vi "PH_PowerUnit_BaseClass.panel.vi"() -> ()   [LabVIEW 2014, in "PH_PowerUnit_BaseClass.lvlib"]
uses:
  PH_PowerUnit_BaseClass.lvlib
  PH_StatusHandler/PH_StatusHandler.GUI element.ctl
  PH_PowerUnit_BaseClass.GUI Refs to pack.ctl
  PH_PowerUnit_BaseClass.GUI Refs.ctl
  CSCore/CSObj/CSObj.lvlib
  PH_Common/PH_Common.lvlib
  PH_Class/PH_Class.lvlib
  PH_StatusHandler/PH_StatusHandler.lvlib
panel:
  out "Timing":u32(colorbox)=6618880
  in  "PU on":bool
  out "Seq SM State":string
  out "PSDB Status":u32(colorbox)=6618880 caption="PSDB"
  out "Dummy 2":u32(colorbox)=6618880
  out "Status":T1 caption="State PU"
  out "Dummy 1":u32(colorbox)=6618880
  in  "Exit":bool
  out "Waiting Time":dbl=999999.0
  out "error out":errorcluster
  in  "Delete":bool
  in  "error in (no error)":errorcluster
  in  "object ref":refnum<vi>
  out "Enabled":u32(colorbox)=6618880
  # "PCS"
  # "3.40"
  # "s"
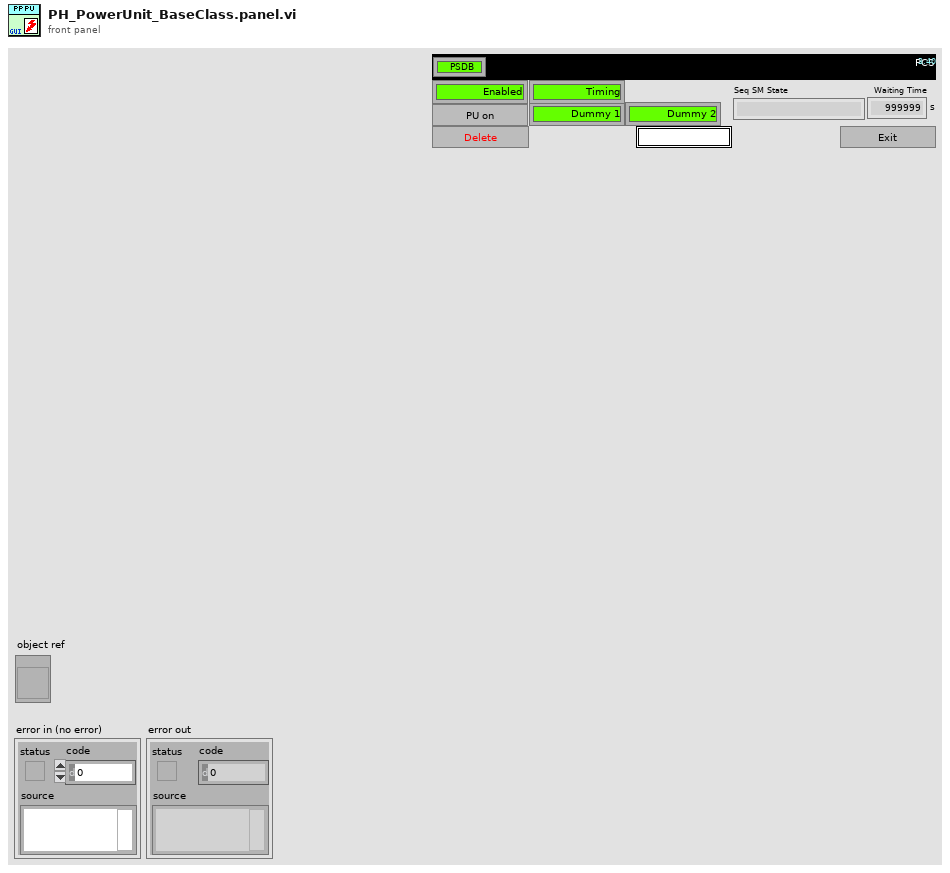
[diagram p1: front panel]
types:
  T1 = typedef "PH_StatusHandler.lvlib/PH_StatusHandler.GUI element.ctl" = u16
  T2 = typedef "PH_PowerUnit_BaseClass.lvlib/PH_PowerUnit_BaseClass.GUI Refs to pack.ctl" = cluster{"GUI Refs":T3, "Enabled":refnum<vi>, "PU on":refnum<vi>, "Waiting Time":refnum<vi>, "Timing.Instance":refnum<vi>, "Seq SM State":refnum<vi>, "Subscribed Trendmssgs":refnum<vi>[]}
  T3 = typedef "PH_PowerUnit_BaseClass.lvlib/PH_PowerUnit_BaseClass.GUI Refs.ctl" = cluster{"Delete Inst":refnum<vi>, "State TO SM":refnum<vi>, "State SM":refnum<vi>, "Fire":refnum<vi>}
  T4 = cluster{"GUI Refs Power Unit Base Class":T2, "PSDB Status":refnum<vi>}
  T5 = typedef "PH_PowerUnit_BaseClass.lvlib/PH_PowerUnit_BaseClass.i attribute.ctl" = cluster{"Constructor finished":bool, "PU":cluster{"In use":bool, "Service ID in use":i32, "GUI Ref":refnum<vi>}, "Enabling":cluster{"State":T6, "GUI Ref":refnum<vi>}, "Timing":cluster{"Last Shot":dbl, "Time between Shots [Sec]":dbl, "Waiting Time over?":bool, "Service ID Waiting Time":i32, "GUI Ref":refnum<vi>, "Instance":cluster{"Status":T7, "linked?":bool, "GUI Ref":refnum<vi>}}, "Sequencer":cluster{"SM State":string, "GUI Ref":refnum<vi>, "linked":bool}, "Subscribed Trendmssgs":cluster{"Tagname":string, "Status":T7, "linked?":bool, "Shot Condition":T7, "GUI Ref":refnum<vi>}[], "PP PU":T8, "Default Voltage (V)":dbl, "GUI Refs":T3, "PSDB data":cluster{"Shot Voltage [V]":dbl, "State TO SM":T9, "Write 2 early":bool}, "State TO SM":T9}
  T6 = typedef "PH_SystemInformation.lvlib/PH_SystemInformationEnabling State.ctl" = i32
  T7 = typedef "PH_StatusHandler.lvlib/PH_StatusHandler.Status.ctl" = i16
  T8 = typedef "PH_PP_Common.lvlib/PH_PP_Common.PUs.ctl" = enum16{"no Info", "PA-19mm-1", "PA-19mm-2", "PA-45mm-PILC", "PA-45mm-MAIN", "MA-PU-1", "MA-PU-2", "MA-PU-3", "MA-PU-4", "MA-PU-5", "MA-PU-6", "MA-FR", "MA-PILC", "PA-45mm-DP"}
  T9 = typedef "PH_PowerUnit_BaseClass.lvlib/PH_PowerUnit_BaseClass.SM States.ctl" = enum16{".", "Stand by", "Switch PU on", "Configure", "Set Default Voltage", "Set STANDBY", "Set READY", "Wait for Shot Cmd", "Open Dump Rods", "Open Ross Relais", "Close Ross Relais", "Switch PSU on", "Switch PSU off", "Charge", "Switch GD Channel on", "Close Dump Rods", "Rods-TO", "RR-TO", "PSU-TO", "Trigger-TO"}
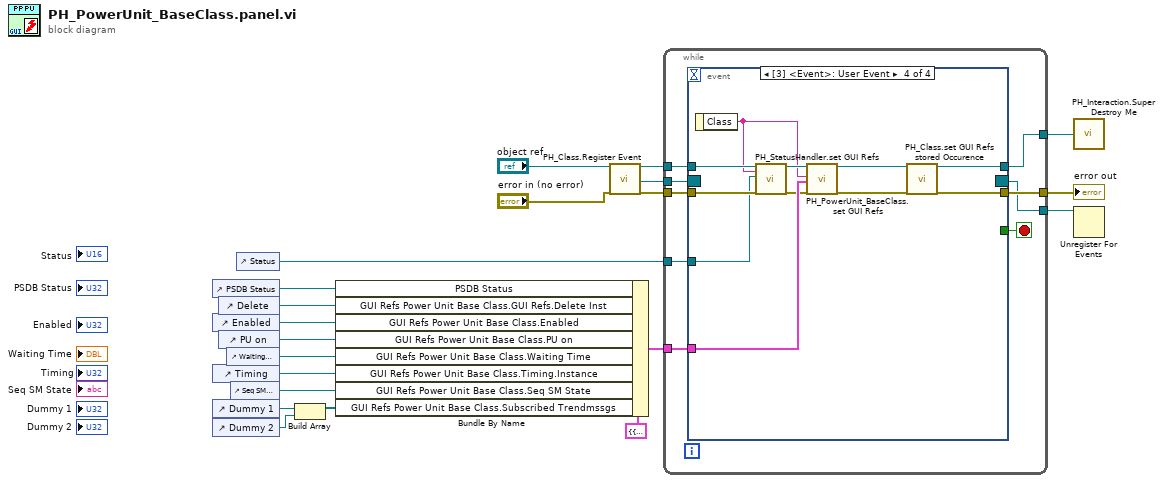
[diagram p0: block diagram]
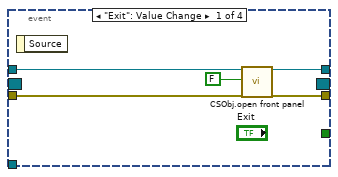
[diagram p2: hidden frame]
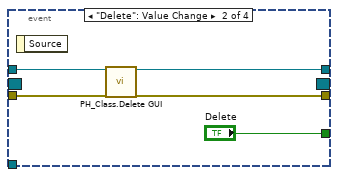
[diagram p3: hidden frame]
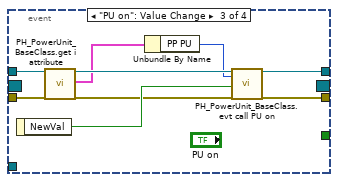
[diagram p4: hidden frame]
diagram:
  n1 = control-ref of="PSDB Status"() -> (w12:refnum<vi>)
  n2 = control-ref of="Enabled"() -> (w10:refnum<vi>)
  n3 = control-ref of="Timing"() -> (w7:refnum<vi>)
  n4 = control-ref of="Dummy 1"() -> (w19:refnum<vi>)
  n5 = control-ref of="Dummy 2"() -> (w18:refnum<vi>)
  n6 = control-ref of="Delete"() -> (w11:refnum<vi>)
  n7 = control-ref of="PU on"() -> (w9:refnum<vi>)
  n8 = control-ref of="Waiting Time"() -> (w8:refnum<vi>)
  n9 = control-ref of="Seq SM State"() -> (w6:refnum<vi>)
  n10 = control-ref of="Status"() -> (w1:refnum<vi>)
  n11 = Build Array(w19, w18) -> (w5:refnum<vi>[])
  n12 = Bundle By Name(cluster=T4 {"GUI Refs Power Unit Base Class"={"GUI Refs"={"Delete Inst"=refnum, "State TO SM"=refnum, "State SM"=refnum, "Fire"=refnum}, "Enabled"=refnum, "PU on"=refnum, "Waiting Time"=refnum, "Timing.Instance"=refnum, "Seq SM State"=refnum, "Subscribed Trendmssgs"=[]}, "PSDB Status"=refnum} ("GUI Refs"), "PSDB Status"=w12, "GUI Refs Power Unit Base Class.GUI Refs.Delete Inst"=w11, "GUI Refs Power Unit Base Class.Enabled"=w10, "GUI Refs Power Unit Base Class.PU on"=w9, "GUI Refs Power Unit Base Class.Waiting Time"=w8, "GUI Refs Power Unit Base Class.Timing.Instance"=w7, "GUI Refs Power Unit Base Class.Seq SM State"=w6, "GUI Refs Power Unit Base Class.Subscribed Trendmssgs"=w5) -> (w2:T4)
  n13 = call "PH_Class.Register Event.vi"("i ref in"="object ref", "error in (no error)"="error in (no error)") -> ("i ref out"=w17:refnum<vi>, "Event Registration Refnum"=w15:refnum<event-registration>, "error out"=w16:errorcluster)  [unwired: 15 in]
  n14 = while {
    tunnel: w17 -> [w27]
    tunnel: [w26] -> w20
    tunnel: w16 -> [w29]
    tunnel: [w28] -> w21
    tunnel: w15 -> [w25]
    tunnel: [w24] -> w14
    tunnel: w2 -> [w23]
    tunnel: w1 -> [w22]
    stop <- w30 stop-if-true
    n15 = event shown="[3] <Event>: User Event" {
      selector: w25 -> [_ _ _ _]
      dyn-events: [_ _ _ _] -> w24
      timeout: _ -> [_ _ _ _]
      tunnel: [_ "Delete" _ _] -> w30
      tunnel: w27 -> [w32 w39 w44 w53]
      tunnel: w29 -> [w35 w38 w48 w57]
      tunnel: [w34 w36 w47 w59] -> w28
      tunnel: [w31 w37 w46 w60] -> w26
      tunnel: w23 -> [_ _ _ w55]
      tunnel: w22 -> [_ _ _ w50]
      event "Exit": Value Change {
        n16 = event-data() -> ()  [unwired: 1 in, 1 out]
        n17 = call "CSObj.open front panel.vi"("i ref in"=w32, "frontPanelOpen"=FALSE ("front panel open"), "error in (no error)"=w35) -> ("i ref out"=w31:refnum<vi>, "error out"=w34:errorcluster)  [unwired: 15 in]
      }
      event "Delete": Value Change {
        n18 = event-data() -> ()  [unwired: 1 in, 1 out]
        n19 = call "PH_Class.Delete GUI.vi"("VI in"=w39, "error in (no error)"=w38) -> ("VI out"=w37:refnum<vi>, "error out"=w36:errorcluster)  [unwired: 16 in]
      }
      event "PU on": Value Change {
        n20 = event-data() -> ("NewVal"=w49:bool)  [unwired: 1 in]
        n21 = call "PH_PowerUnit_BaseClass.get i attribute.vi"("i ref in"=w44, "error in (no error)"=w48) -> ("i ref out"=w43:refnum<vi>, "i attribute"=w42:T5, "error out"=w45:errorcluster)  [unwired: 15 in]
        n22 = Unbundle By Name(w42) -> ("PP PU"=w41:T8)
        n23 = call "PH_PowerUnit_BaseClass.evt call PU on.vi"("i ref in"=w43, "PowerUnit"=w41, "PU on"=w49, "error in (no error)"=w45) -> ("i ref out"=w46:refnum<vi>, "error out"=w47:errorcluster)  [unwired: 14 in]
      }
      event User Event {
        n24 = event-data() -> ("Class"=w51:string)  [unwired: 1 in]
        n25 = call "PH_StatusHandler.set GUI Refs.vi"("i ref in"=w53, "Class"=w51, "GUI Ref"=w50, "error in (no error)"=w57) -> ("i ref out"=w52:refnum<vi>, "error out"=w54:errorcluster)  [unwired: 14 in]
        n26 = call "PH_PowerUnit_BaseClass.set GUI Refs.vi"("i ref  in"=w52, "Class"=w51, "GUI Refs"=w55, "error in"=w54) -> ("i ref out"=w58:refnum<vi>, "error out"=w56:errorcluster)  [unwired: 14 in]
        n27 = call "PH_Class.set GUI Refs stored Occurence.vi"("i ref in"=w58, "error in (no error)"=w56) -> ("i ref out"=w60:refnum<vi>, "error out"=w59:errorcluster)  [unwired: 16 in]
      }
    }
  }
  "error out" <- w21
  n28 = call "PH_Interaction.Super Destroy Me.vi"("i ref out"=w20) -> ()
  n29 = Unregister For Events(event registration refnum=w14) -> ()  [unwired: 1 in, 1 out]
